vi "LockSplitters.vi"(8 "error in":errorcluster, 10 "Splitter Position Locked":bool=TRUE, 11 "Splitters":T1) -> (0 "error out":errorcluster)   [LabVIEW 2022 SP3, in "PentaPanesLibrary.lvlib" / "PentaPanes.lvclass"]
uses:
  PentaPanes.lvclass
  SplittersCluster.ctl
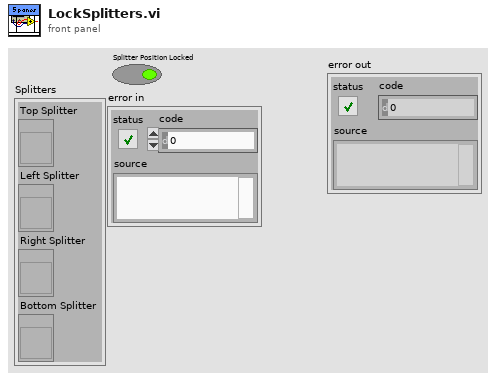
[diagram p1: front panel]
types:
  T1 = typedef "PentaPanesLibrary.lvlib/PentaPanes.lvclass/SplittersCluster.ctl" = cluster{"Top Splitter":refnum<vi>, "Left Splitter":refnum<vi>, "Right Splitter":refnum<vi>, "Bottom Splitter":refnum<vi>}
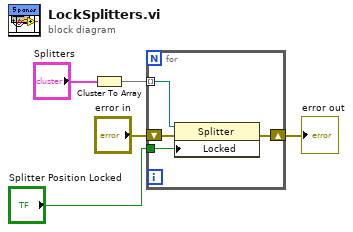
[diagram p0: block diagram]
diagram:
  n1 = Cluster To Array(cluster="Splitters") -> (array=w5:refnum<vi>[])
  n2 = for {
    tunnel: w5 -> [w9] mode=indexing
    tunnel: "Splitter Position Locked" -> [w8]
    shift-right: [w6] -> w1
    shift-left: "error in" -> [w7]
    n3 = property class="Splitter"(reference=w9, error in=w7, "Locked"=w8) -> (error out=w6:errorcluster)  [unwired: 1 out]
  }
  "error out" <- w1
